vi "Get Picture Solution.vi"(8 "error in (no error)":errorcluster, 11 "Grassfire 2D In":refnum<class "Grassfire 2D.lvclass">) -> (0 "error out":errorcluster, 2 "2D Picture":picture, 3 "Grassfire 2D Out":refnum<class "Grassfire 2D.lvclass">)   [LabVIEW 2019, in "Grassfire 2D.lvclass"]
uses:
  Grassfire 2D.lvclass
  Grassfire 2D.lvclass/Grassfire 2D.ctl
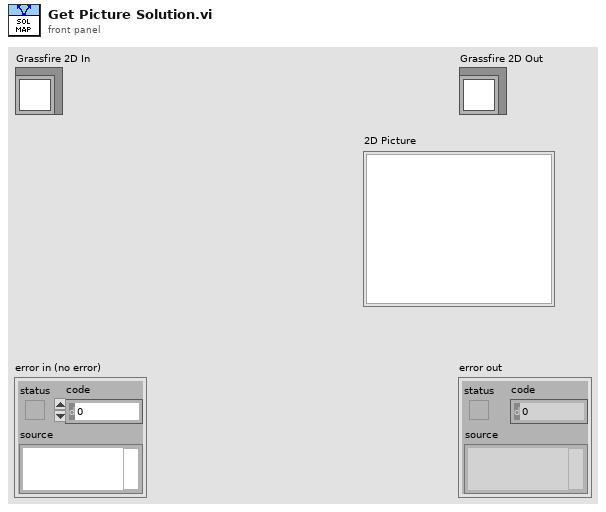
[diagram p1: front panel]
types:
  T1 = typedef "Grassfire 2D.lvclass/Node Address--cluster.ctl" = cluster{"Row":i32, "Column":i32}
  T2 = typedef "Grassfire 2D.lvclass/Node Value--cluster.ctl" = cluster{"Type":T3, "Distance":i32}
  T3 = typedef "Shared.lvlib/Node Type--enum.ctl" = enum16{"Empty", "Blocked", "Start", "End", "Path"}
  T4 = typedef "imagedata.ctl" = cluster{"image type":i32, "image depth":i32, "image":u8[], "mask":u8[], "colors":u32[], "Rectangle":cluster{"left":i16, "top":i16, "right":i16, "bottom":i16}}
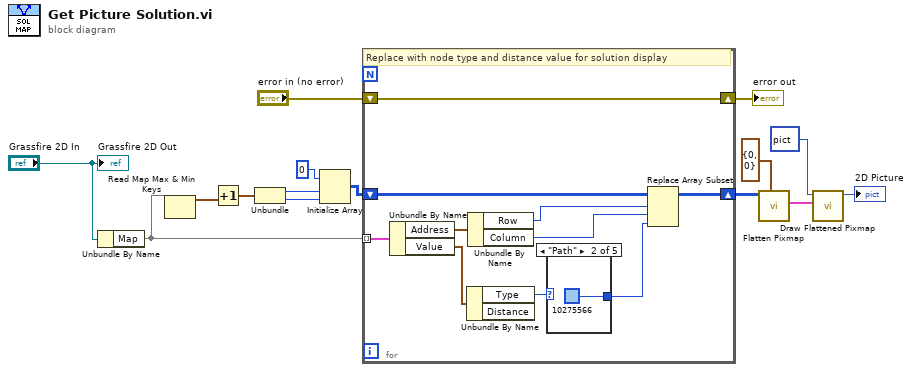
[diagram p0: block diagram]
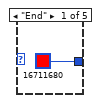
[diagram p2: hidden frame]
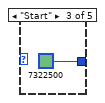
[diagram p3: hidden frame]
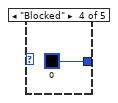
[diagram p4: hidden frame]
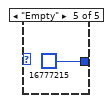
[diagram p5: hidden frame]
diagram:
  n1 = Unbundle By Name("Grassfire 2D In") -> ("Map"=w14:map{T1, T2})
  n2 = Read Map Max & Min Keys(11:w14) -> (3:w10:T1)  [unwired: 1 out]
  n3 = Increment(x=w10) -> (x+1=w9:T1)
  n4 = Unbundle(w9) -> ("Row"=w8:i32, "Column"=w7:i32)
  n5 = Initialize Array(u32 0, w8, w7) -> (w15:u32[][])
  n6 = for {
    shift-right: [w24] -> w1
    shift-left: w15 -> [w25]
    tunnel: w14 -> [w22] mode=indexing
    shift-right: [w23] -> w11
    shift-left: "error in (no error)" -> [w23]
    # "Replace with node type and distance value for solution display"
    n7 = Unbundle By Name(w22) -> ("Address"=w20:T1, "Value"=w21:T2)
    n8 = Unbundle By Name(w21) -> ("Type"=w17:T3)  [unwired: 1 out]
    n9 = Unbundle By Name(w20) -> ("Row"=w19:i32, "Column"=w18:i32)
    n10 = case shown="\"Path\"" w17 {
      tunnel: [u32 16711680 ("Pen Color") u32 10275566 ("Pen Color") u32 7322500 ("Pen Color") u32 0 ("Pen Color") u32 16777215 ("Pen Color")] -> w16
      frame "End" {
      }
      frame "Path" {
      }
      frame "Start" {
      }
      frame "Blocked" {
      }
      frame "Empty" {
      }
    }
    n11 = Replace Array Subset(array=w25, new element=w16, index (row)=w19, index (col)=w18) -> (w24:u32[][])
  }
  "error out" <- w11
  n12 = call <vilib>:"Flatten Pixmap.vi"("top left"=cluster{"x":i16, "y":i16} {"x"=0, "y"=0}, "24-bit pixmap"=w1) -> ("image data"=w4:T4)  [unwired: 9 in]
  n13 = call <vilib>:"Draw Flattened Pixmap.vi"("image data"=w4, "picture"=picture data[5B]) -> ("new picture"=→"2D Picture":picture)  [unwired: 7 in]
  "Grassfire 2D Out" <- "Grassfire 2D In"
